vi "Main_08A.vi"() -> ()   [LabVIEW 2024]
uses:
  Map_Antena.ctl
  Cluster_Position.ctl
  <vilib>/Utility/miscctls.llb/LVMapReplaceAction.ctl
panel:
  out "final":string[][](array[string])
  out "Antena Map":T1
  out "2D Array":string[][](array[string])
  in  "Use Puzzle":bool
  out "Answer":u32
  in  "Puzzle":string="............s...............1.....................\n......................E......3.....S..............\n.......................3.....S....................\n...e........T.t.......S.1...........I.............\n..................B..................I.....O......\ng.......z........i39......B..I....................\n.......s....S.......3......................i..I...\n....e.............2..........B....................\n.......tC...z.......g......1......................\n.E......s....R....................................\n..G...t..........2................................\n.........K...C.......2............................\n....T..e...........5...C..........................\n...T................................O...o.........\n...............................g..............o...\n.........z...................g......i............o\n...9.E............H...........Y.......O...........\n..........R..H...............7.O..................\n...........H.............v......7........B........\n..9.Q.......................W......1........Y.....\n.........................z.7.................Y....\n.....Q................................v...........\n....K.......E.....R...............2..........o....\n.n............H......v...........................Y\n.G.y..........................Q...................\n......G....A5.....................h...............\n..........D...5.w...9.............................\n......n....5...L..................................\n............................v.....................\n............L...0t..........7.....................\n..n....k............y....................W........\n..k..........0.........................W..........\n...n.......R..L..a........................W.......\n.........................................h........\n..0..L........c...b...............................\n.....................8.y..........................\n.......w.................6.............h.......N..\n..........y..4....................................\n...0....8...k.....Z........r......................\n..............a...8Z.........G......4.............\n........4..b.q.....................K..............\n.q...........kZ.K......b..D.........d.............\n.8.....................D................r.........\n.....w.........a...............d........A.........\n................................d.A.hV............\n................c..........D.....V....r...........\n.......Z......6.....l........................A.d..\n...................l..6..c....b......r...........N\n......a....4........q..l..V..c................N...\nl.....w...........q..6............V..............."
  in  "Example":string="............\n........0...\n.....0......\n.......0....\n....0.......\n......A.....\n............\n............\n........A...\n.........A..\n............\n............"
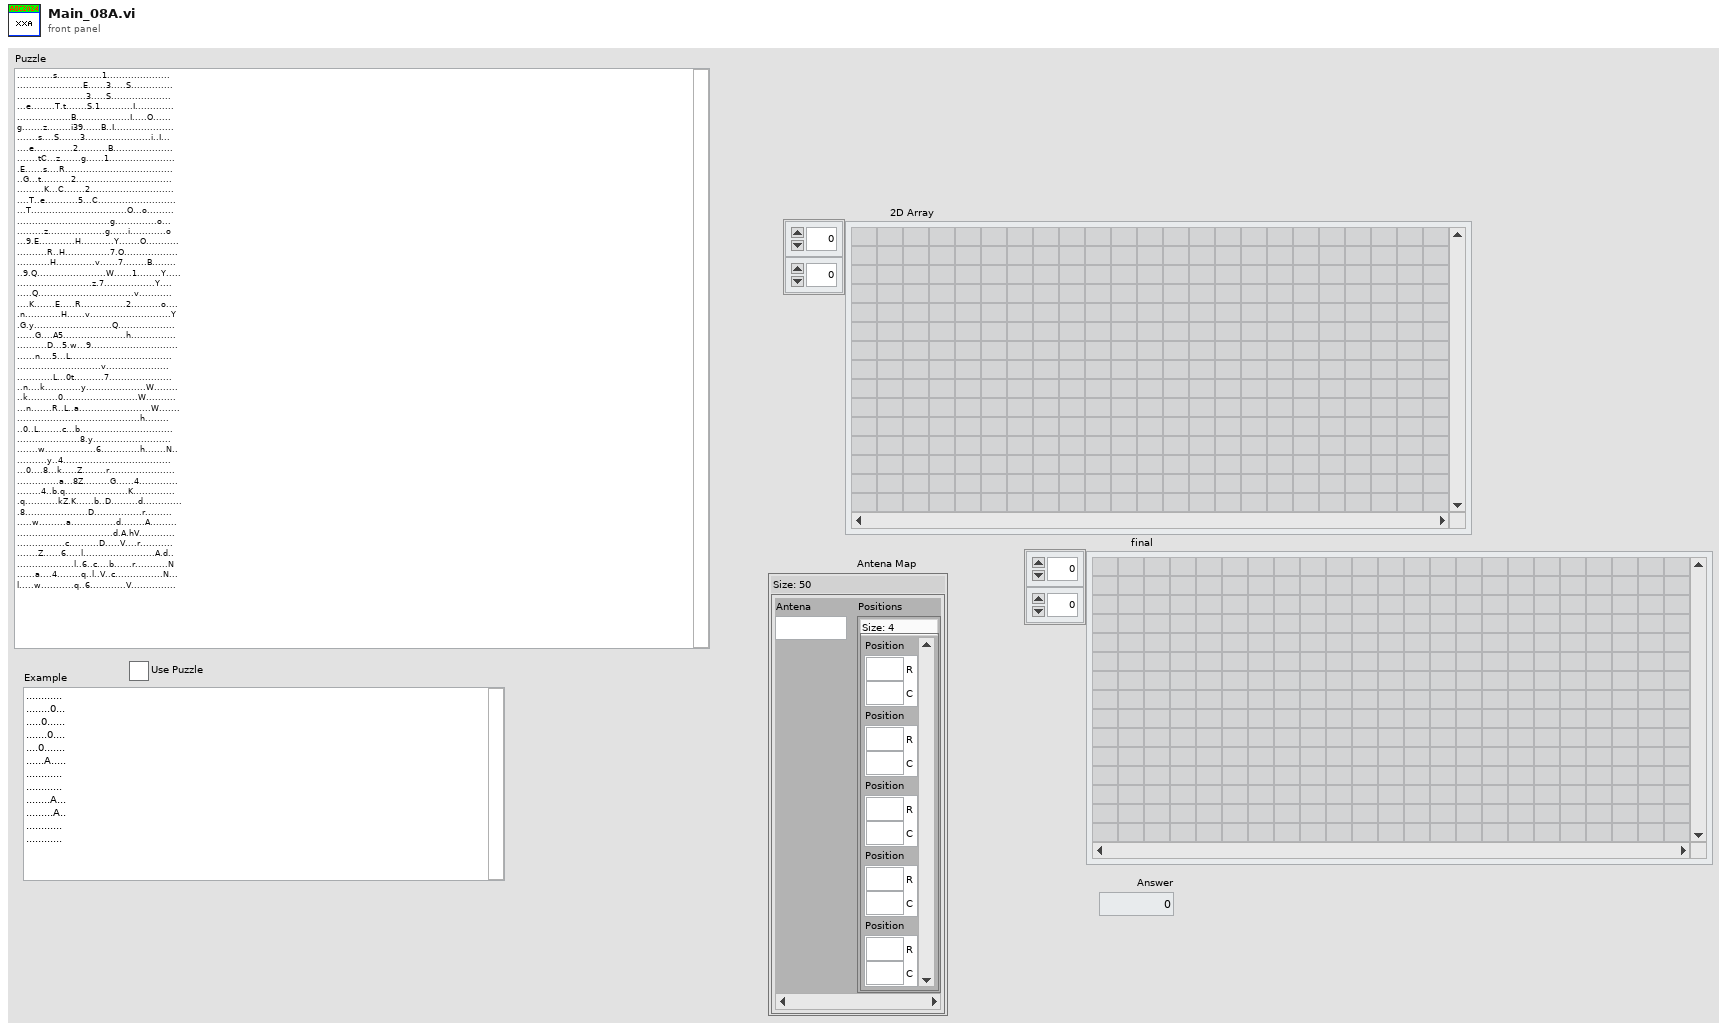
[diagram p1: front panel]
types:
  T1 = typedef "Map_Antena.ctl" = map{string, set{T2}}
  T2 = typedef "Cluster_Position.ctl" = cluster{"R":i32, "C":i32}
  T3 = typedef "LVMapReplaceAction.ctl" = enum32{"Modify Entry only if found", "Add or Modify Entry", "Delete Entry"}
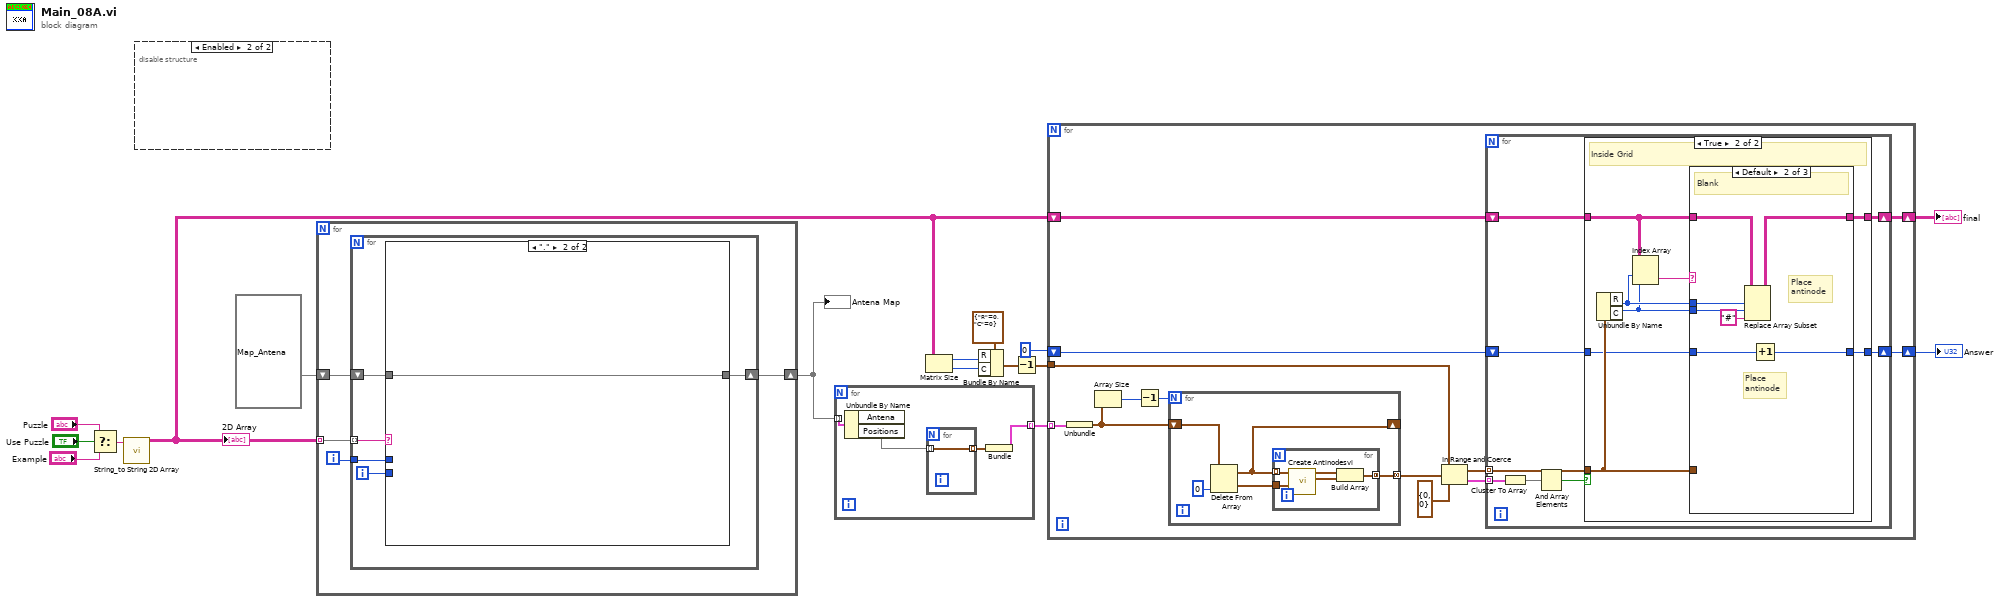
[diagram p0: block diagram]
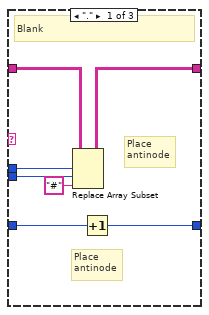
[diagram p3: hidden frame]
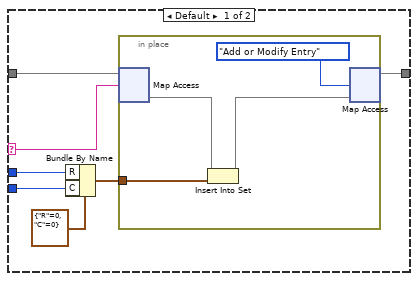
[diagram p5: hidden frame]
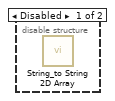
[diagram p6: hidden frame]
diagram:
  n1 = Select(t="Puzzle", s="Use Puzzle", f="Example") -> (s? t:f=w13:string)
  n2 = call "String_to String 2D Array.vi"("Input String"=w13) -> ("2D Array"=w4:string[][])  [unwired: 10 in]
  "2D Array" <- w4
  n3 = disable-structure shown="Enabled" {
    frame Disabled {
      n4 = call "String_to String 2D Array.vi"() -> ()  [unwired: 11 in, 1 out]
    }
    frame Enabled {
    }
  }
  n5 = for {
    tunnel: w4 -> [w20] mode=indexing
    shift-right: [w18] -> w11
    shift-left: T1 {} ("Antena Map") -> [w19]
    i -> [w17]
    n6 = for {
      tunnel: w20 -> [w25] mode=indexing
      shift-right: [w21] -> w18
      shift-left: w19 -> [w24]
      tunnel: w17 -> [w23]
      i -> [w22]
      n7 = case shown="\".\"" w25 {
        selector: w25 -> [w31 _]
        tunnel: w24 -> [w32 w37]
        tunnel: w23 -> [w29 _]
        tunnel: w22 -> [w28 _]
        tunnel: [w26 w37] -> w21
        frame Default {
          n8 = Bundle By Name(cluster=T2 {"R"=0, "C"=0} ("Position"), "R"=w29, "C"=w28) -> (w27:T2)
          n9 = in-place {
            in-place-border: w27 -> [w33]
            n10 = in-place-map #1(w32, w31) -> (w35:set{T2})  [unwired: 1 in, 1 out]
            n11 = Insert Into Set(10:w33, 11:w35) -> (3:w34:set{T2})  [unwired: 1 out]
            n12 = in-place-map #1(w34, LVMapReplaceAction."Add or Modify Entry" ("action")) -> (w26:T1)  [unwired: 2 out]
          }
        }
        frame "." {
        }
      }
    }
  }
  "Antena Map" <- w11
  n13 = for {
    tunnel: w11 -> [w41] mode=indexing
    tunnel: [w38] -> w10 mode=indexing
    n14 = Unbundle By Name(w41) -> ("Positions"=w40:set{T2})  [unwired: 1 out]
    n15 = for {
      tunnel: w40 -> [w42] mode=indexing
      tunnel: [w42] -> w39 mode=indexing
    }
    n16 = Bundle(w39) -> (w38:cluster{T2[]})  [unwired: 1 in]
  }
  n17 = Matrix Size(0:w4) -> (1:w8:i32, 2:w7:i32)
  n18 = Bundle By Name(cluster=T2 {"R"=0, "C"=0} ("Position"), "R"=w8, "C"=w7) -> (w6:T2)
  n19 = Decrement(x=w6) -> (x-1=w5:T2)
  n20 = for {
    tunnel: w10 -> [w55] mode=indexing
    tunnel: w5 -> [w50]
    shift-right: [w44] -> w2
    shift-left: u32 0 -> [w45]
    shift-right: [w43] -> w1
    shift-left: w4 -> [w46]
    n21 = Unbundle(w55) -> (w54:T2[])
    n22 = Array Size(array=w54) -> (size(s)=w53:i32)
    n23 = Decrement(x=w53) -> (x-1=w52:i32)
    n24 = for {
      N: w52 -> [_]
      shift-right: [w91] -> _
      shift-left: w54 -> [w94]
      tunnel: [w90] -> w51 mode=concatenating
      n25 = Delete From Array(array=w94, index=0) -> (deleted portion=w92:T2, array with subset deleted=w91:T2[])  [unwired: 1 in]
      n26 = for {
        tunnel: w92 -> [w98]
        tunnel: w91 -> [w99] mode=indexing
        tunnel: [w95] -> w90 mode=concatenating
        n27 = call "Create Antinodesvi.vi"("Antena 2"=w98, "Antena 1"=w99) -> ("AntiNode 2 Out"=w96:T2, "AntiNoed 1 Out"=w97:T2)  [unwired: 8 in]
        n28 = Build Array(w97, w96) -> (w95:T2[])
      }
    }
    n29 = In Range and Coerce(upper limit=w50, x=w51, lower limit=T2 {"R"=0, "C"=0}) -> (coerced(x)=w47:T2[], In Range?=w48:cluster{"R":bool, "C":bool}[])
    n30 = for {
      tunnel: w48 -> [w63] mode=indexing
      tunnel: w47 -> [w60] mode=indexing
      shift-right: [w58] -> w43
      shift-left: w46 -> [w59]
      shift-right: [w56] -> w44
      shift-left: w45 -> [w57]
      n31 = Cluster To Array(cluster=w63) -> (array=w62:bool[])
      n32 = And Array Elements(Boolean array=w62) -> (logical AND=w61:bool)
      n33 = case shown="True" w61 {
        tunnel: w60 -> [_ w71]
        tunnel: w59 -> [w65 w72]
        tunnel: [w65 w68] -> w58
        tunnel: w57 -> [w64 w67]
        tunnel: [w64 w66] -> w56
        frame False {
          # "Off Grid"
        }
        frame True {
          # "Inside Grid"
          n34 = Unbundle By Name(w71) -> ("R"=w70:i32, "C"=w69:i32)
          n35 = Index Array(array=w72, index (row)=w70, index (col)=w69) -> (element=w73:string)
          n36 = case shown="Default" w73 {
            tunnel: w72 -> [w80 w87 w89]
            tunnel: w71 -> [_ _ _]
            tunnel: w70 -> [w78 w85 _]
            tunnel: w69 -> [w77 w84 _]
            tunnel: [w79 w86 w89] -> w68
            tunnel: w67 -> [w75 w82 w88]
            tunnel: [w74 w81 w88] -> w66
            frame "." {
              # "Place\nantinode"
              # "Place\nantinode"
              # "Blank"
              n37 = Replace Array Subset(array=w80, new element="#" ("new element/subarray"), index (row)=w78, index (col)=w77) -> (w79:string[][])
              n38 = Increment(x=w75) -> (x+1=w74:u32)
            }
            frame Default {
              # "Place\nantinode"
              # "Place\nantinode"
              # "Blank"
              n39 = Replace Array Subset(array=w87, new element="#" ("new element/subarray"), index (row)=w85, index (col)=w84) -> (w86:string[][])
              n40 = Increment(x=w82) -> (x+1=w81:u32)
            }
            frame "#" {
            }
          }
        }
      }
    }
  }
  "Answer" <- w2
  "final" <- w1
